vi "test2-TestFilterJKISMStringQueueVI.vi"(8 "error in (no error)":errorcluster, 11 "TestCase in":refnum<class "testcase-CSMManagementAPI.lvclass">) -> (0 "error out":errorcluster, 3 "TestCase out":refnum<class "testcase-CSMManagementAPI.lvclass">)   [LabVIEW 2017, in "testcase-CSMManagementAPI.lvclass"]
uses:
  testcase-CSMManagementAPI.lvclass
  src/user.lib/_NEVSTOP/Communicable State Machine(CSM)/AdvanceAPI/CSM - Revert Arguments-Safe String.vi
  src/user.lib/_NEVSTOP/Communicable State Machine(CSM)/_Shared/Trim Single-line Text.vi
  src/user.lib/_NEVSTOP/Communicable State Machine(CSM)/AdvanceAPI/CSM - Make String Arguments Safe.vi
  src/user.lib/_NEVSTOP/Communicable State Machine(CSM)/AdvanceAPI/CSM - Break Down Multiple States String.vi
  src/user.lib/_NEVSTOP/Communicable State Machine(CSM)/AdvanceAPI/CSM - Compact Multiple States.vi
  src/user.lib/_NEVSTOP/Communicable State Machine(CSM)/AdvanceAPI/CSM - Keywords.vi
  src/user.lib/_NEVSTOP/Communicable State Machine(CSM)/_Polymophic/CSM - Filter Interrupt Broadcasts.vi
  src/user.lib/_NEVSTOP/Communicable State Machine(CSM)/_Polymophic/CSM - Filter Status Broadcasts.vi
  src/user.lib/_NEVSTOP/Communicable State Machine(CSM)/_Polymophic/CSM - Filter Broadcasts.vi
  src/user.lib/_NEVSTOP/Communicable State Machine(CSM)/_Polymophic/CSM - Filter Sync Messages.vi
  src/user.lib/_NEVSTOP/Communicable State Machine(CSM)/_Polymophic/CSM - Filter Async without Reply Messages.vi
  src/user.lib/_NEVSTOP/Communicable State Machine(CSM)/_Polymophic/CSM - Filter Async Messages.vi
  src/user.lib/_NEVSTOP/Communicable State Machine(CSM)/_Polymophic/CSM - Filter Messges.vi
  src/user.lib/_NEVSTOP/Communicable State Machine(CSM)/_Polymophic/CSM - Filter Local States.vi
  src/user.lib/_NEVSTOP/Communicable State Machine(CSM)/_Polymophic/CSM - Filter Duplicated Lines.vi
  src/user.lib/_NEVSTOP/Communicable State Machine(CSM)/AdvanceAPI/CSM - Filter Messages to Non-Existing Modules.vi
  <vilib>/addons/_JKI Toolkits/VI Tester/TestCase.llb/TestCase.lvclass
  src/user.lib/_NEVSTOP/Communicable State Machine(CSM)/Communicable State Machine.lvlib
  C:/Program Files (x86)/National Instruments/LabVIEW 2017/vi.lib/addons/_JKI Toolkits/VI Tester/TestCase.llb/TestCase.lvclass
panel:
  out "Filter Duplicate Lines No Comments":bool
  out "Filter Duplicate Lines":bool
  out "Filter Duplicate States(Regardless of async/sync/status/interrupt)":bool
  out "Fiter Interrupt Broadcast":bool
  out "Fiter Status Broadcast":bool
  out "Fiter Broadcasts":bool
  out "Filter Messages To Non Existing CSMs":bool
  out "Filter Sync Messages":bool
  out "Filter Async Messages Without Reply":bool
  out "Filter Async Messages":bool
  out "Filter All Messages":bool
  out "Fiter Local States":bool
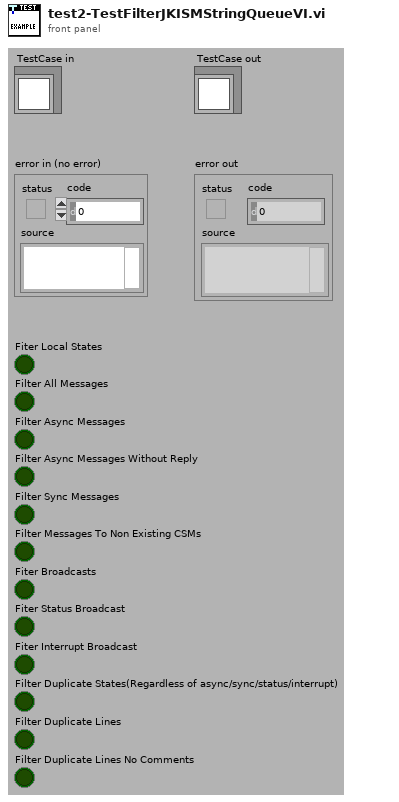
[diagram p1: front panel]
types:
  T1 = enum32{"Invalid", "Standard", "Closed", "Hidden", "Minimized", "Maximized"}
  T2 = enum32{"invalid app kind", "Development System", "Run Time System", "Student Edition", "Embedded LabVIEW", "Evaluation", "Custom"}
  T3 = typedef "Communicable State Machine.lvlib/_CSM_Response Source Message.ctl" = cluster{"‘State":string, "’Arguments":string, "’Error":errorcluster}
  T4 = cluster{"Current VI Reference":refnum<vi>, "Close Panel on Exit?":bool}
  T5 = cluster{"Core":cluster{"Current VI Reference":refnum<vi>, "Close Panel on Exit?":bool}, "Your Boolean data":bool, "Your string data":string}
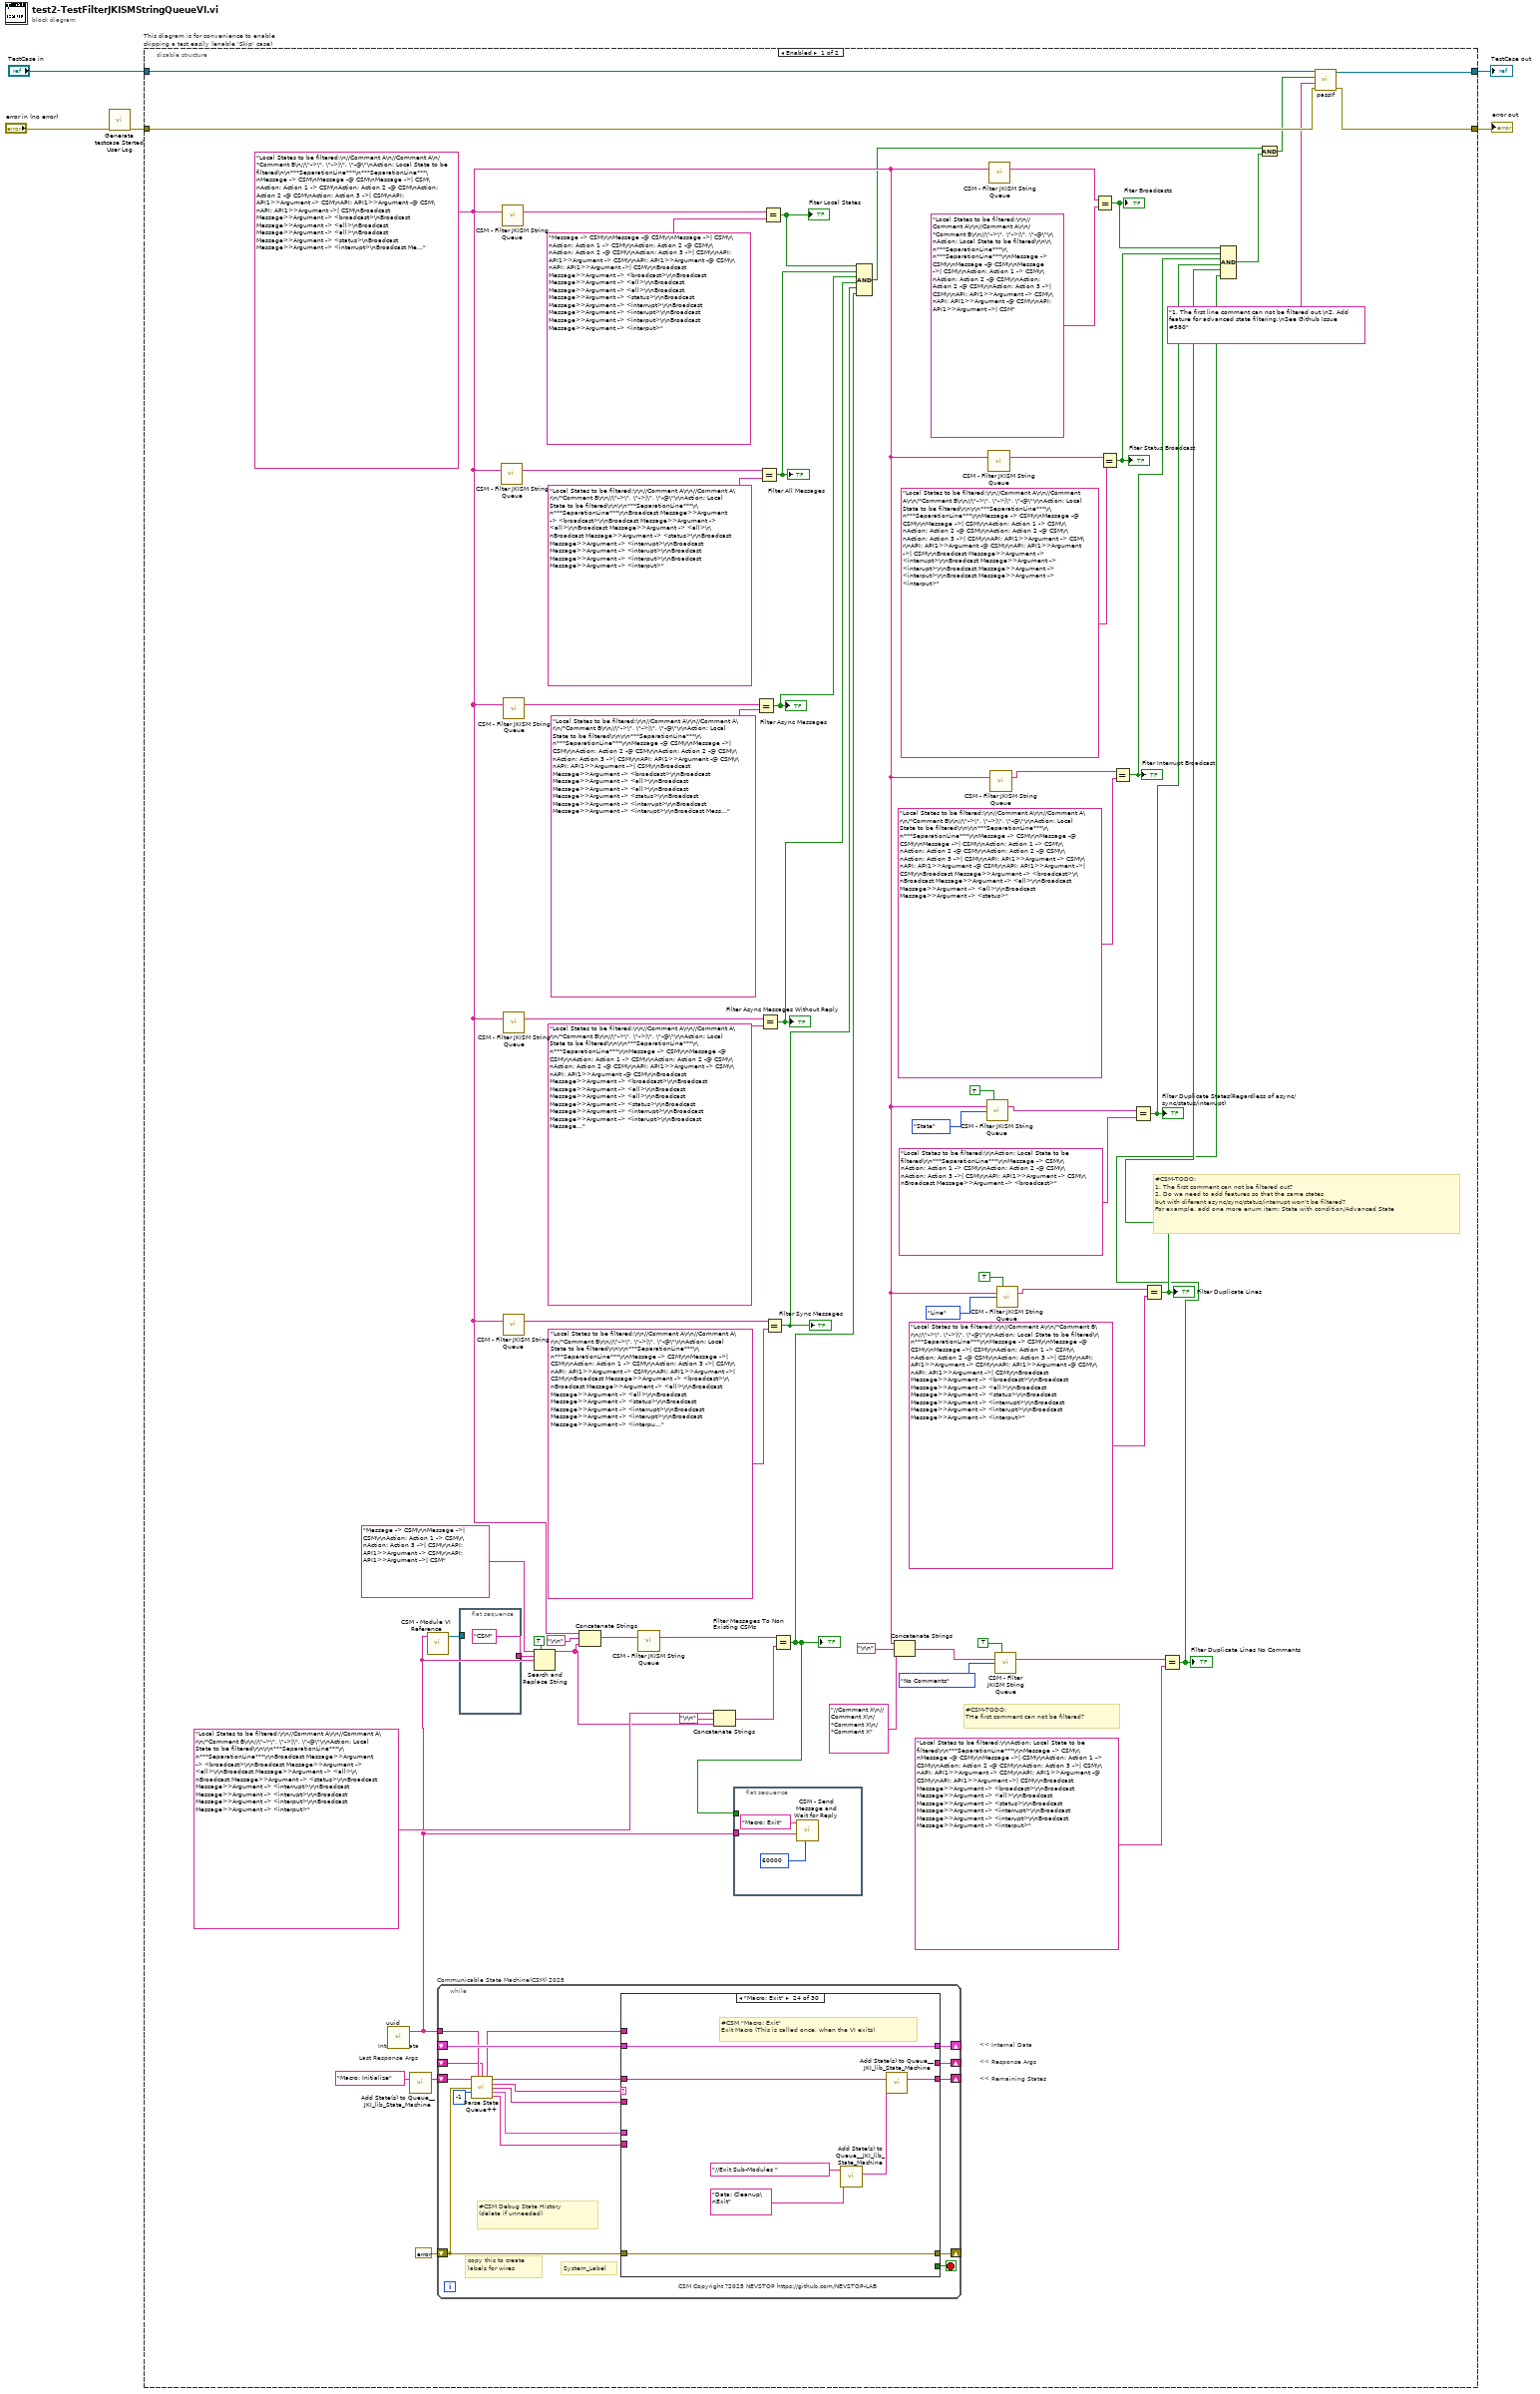
[diagram p0: block diagram]
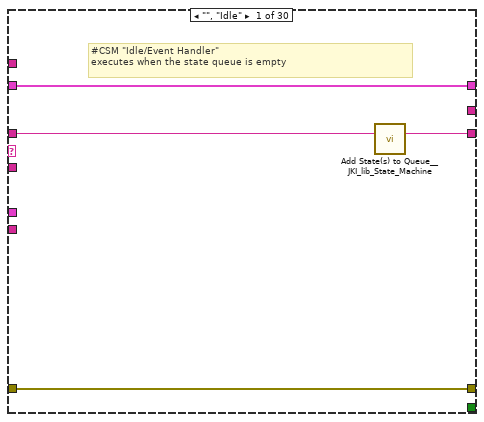
[diagram p2: hidden frame]
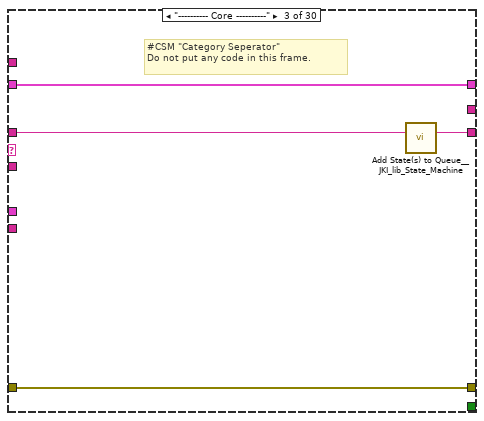
[diagram p4: hidden frame]
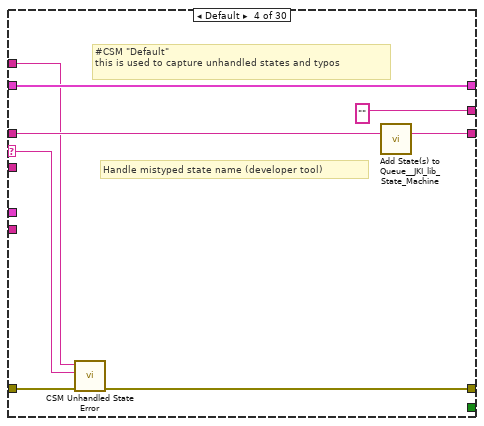
[diagram p5: hidden frame]
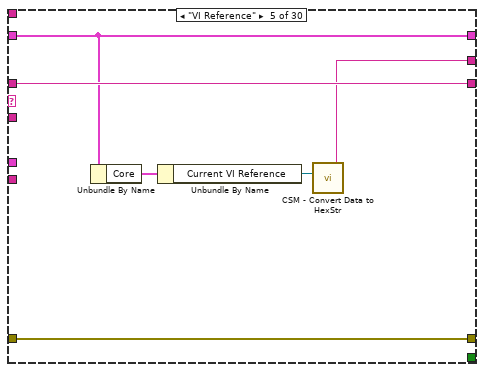
[diagram p6: hidden frame]
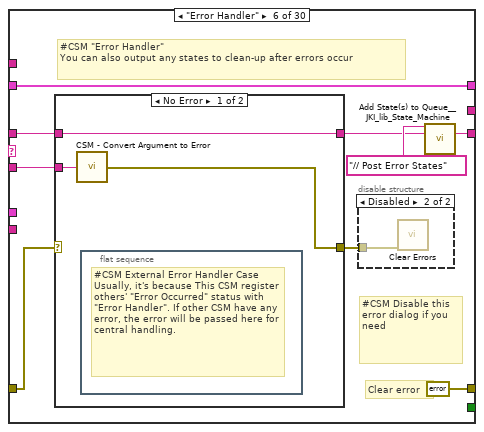
[diagram p7: hidden frame]
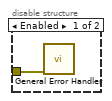
[diagram p8: hidden frame]
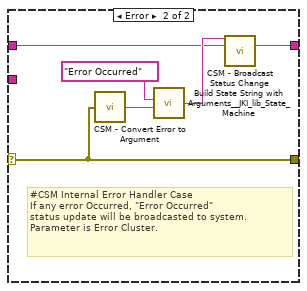
[diagram p9: hidden frame]
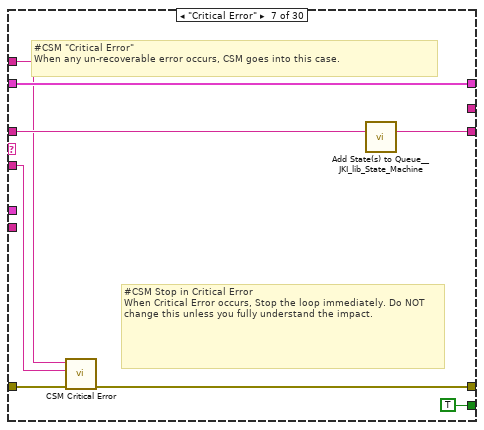
[diagram p10: hidden frame]
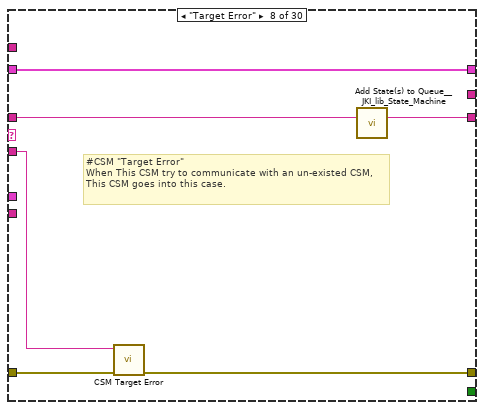
[diagram p11: hidden frame]
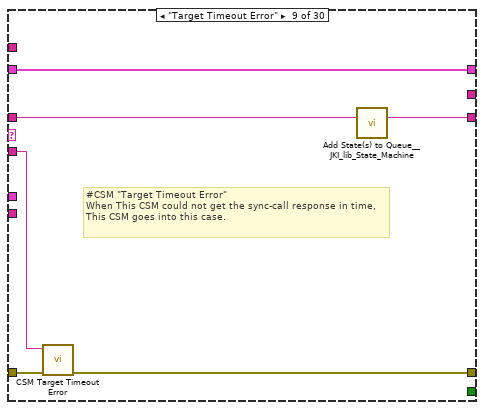
[diagram p12: hidden frame]
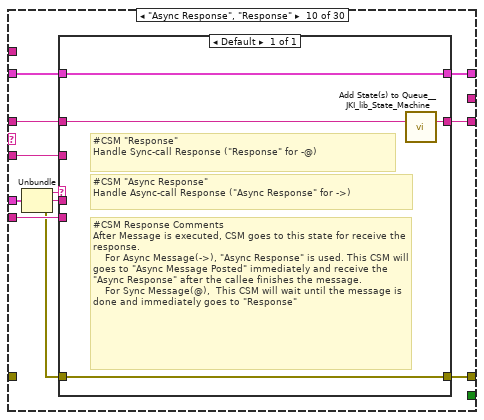
[diagram p13: hidden frame]
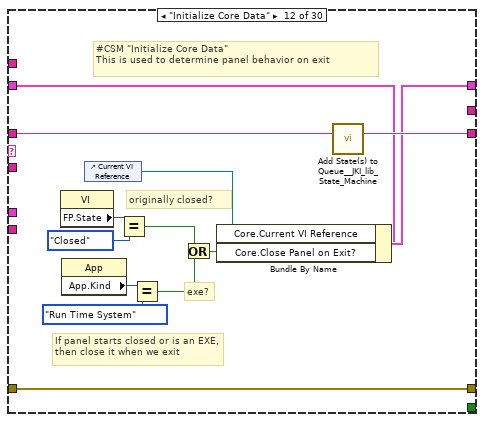
[diagram p15: hidden frame]
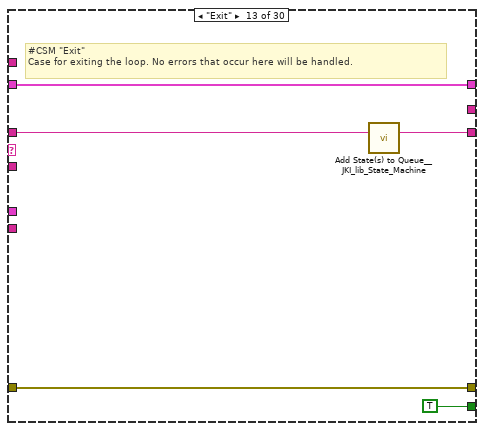
[diagram p16: hidden frame]
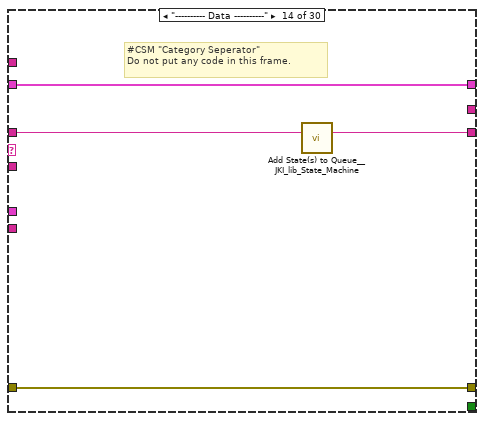
[diagram p17: hidden frame]
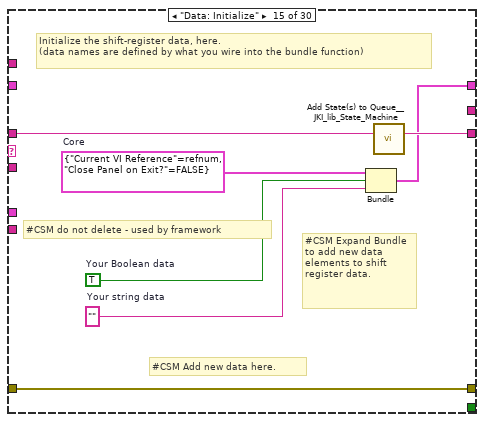
[diagram p18: hidden frame]
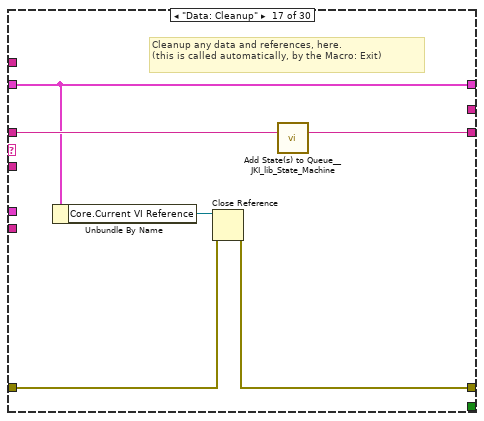
[diagram p20: hidden frame]
diagram:
  n1 = call "Generate testcase Started User Log.vi"("Error In"="error in (no error)") -> ("error out"=w1:errorcluster)  [unwired: 10 in]
  n2 = disable-structure "This diagram is for convenience to enable skipping a test easily (enable 'Skip' case)" shown="Enabled" {
    disable-tunnel: "TestCase in" -> [w32 w354]
    disable-tunnel: [w33 w352] -> w2
    disable-tunnel: [w30 w353] -> w4
    disable-tunnel: w1 -> [w31 w351]
    frame Enabled {
      w38 = "Local States to be filtered:\n//Comment A\n//Comment A\n/*Comment B\n//\"->\", \"->|\", \"-@\"\nAction: Local State to be filtered\n\n***SeparationLine***\n***SeparationLine***\nMessage -> CSM\nMessage -@ CSM\nMessage ->| CSM\nAction: Action 1 -> CSM\nAction: Action 2 -@ CSM\nAction: Action 2 -@ CSM\nAction: Action 3 ->| CSM\nAPI: API1>>Argument -> CSM\nAPI: API1>>Argument -@ CSM\nAPI: API1>>Argument ->| CSM\nBroadcast Message>>Argument -> <broadcast>\nBroadcast Message>>Argument -> <all>\nBroadcast Message>>Argument -> <all>\nBroadcast Message>>Argument -> <status>\nBroadcast Message>>Argument -> <interrupt>\nBroadcast Message>>Argument -> <interupt>\nBroadcast Message>>Argument -> <interput>\nBroadcast Message>>Argument -> <interput>" ("States In")
      # "Last Response Args"
      # "Internal Data"
      # "<< Internal Data"
      # "<< Response Args"
      # "<< Remaining States"
      # "#CSM-TODO:\nTHe first comment can not be filtered?"
      # "#CSM-TODO:\n1. The first comment can not be filtered out?\n2. Do we need to add features so that the same states \nbut with diferent async/sync/status/interrupt won't be filtered?\nFor example, add one more enum item: State with condition/Advanced State"
      n3 = call "uuid.vi"() -> ("UUID"=w7:string)  [unwired: 11 in]
      n4 = call <vilib>:"Add State(s) to Queue__JKI_lib_State_Machine.vi"("State(s) in (\"\")"="Macro: Initialize" ("Init State(\"Macro: Initialize\")")) -> ("States Out"=w11:string)  [unwired: 14 in]
      n5 = call "CSM - Module VI Reference.vi"("CSM Name"=w7) -> ("CSM Module VIRef"=w8:refnum<vi>)  [unwired: 9 in, 1 out]
      n6 = while "Communicable State Machine(CSM) 2025" {
        shift-right: [w88] -> _
        shift-left: _ -> [w87]
        shift-right: [w91] -> _
        shift-left: errorcluster {"status"=FALSE, "code"=0, "source"=""} ("error out") -> [w86]
        shift-right: [w90] -> _
        shift-left: w11 -> [w92]
        tunnel: w7 -> [w84]
        shift-right: [w85] -> _
        shift-left: _ -> [w78]
        stop <- w89 stop-if-true
        # "#CSM Debug State History\n(delete if unneeded)"
        # "copy this to create labels for wires"
        # "System_Label"
        # "CSM Copyright ?2025 NEVSTOP https://github.com/NEVSTOP-LAB"
        n7 = call "Parse State Queue++.vi"("State Queue"=w92, "Name (\"\" to Use UUID)"=w84, "Response Arguments"=w78, "Previous Error"=w86, "Dequeue (1 ms)"=-1 ("Timeout")) -> ("Name Used"=w79:string, "Remaining States"=w93:string, "Current State"=w83:string, "Arguments"=w82:string, "Additional Information"=w81:T3, "Source CSM"=w80:string)  [unwired: 5 in]
        n8 = case shown="\"Macro: Exit\"" w83 {
          selector: w83 -> [_ _ _ w107 _ _ _ _ _ _ _ _ _ _ _ _ _ _ _ _ _ _ _ _ _ _ _ _ _ _]
          tunnel: w93 -> [w94 w99 w104 w111 w117 w123 w144 w150 w156 w164 w175 w189 w194 w198 w205 w207 w214 w218 w222 w228 w243 w312 w317 w324 w326 w330 w335 w342 w346 w350]
          tunnel: w82 -> [_ _ _ _ _ w122 w140 w149 w154 w163 _ _ _ _ _ _ _ _ _ w223 w237 _ _ _ _ _ w333 _ _ _]
          tunnel: w87 -> [w95 w98 w101 w109 w116 w126 w145 w151 w157 w166 w174 w182 w192 w195 _ w206 w209 w215 w220 w226 w239 w309 w314 w321 w325 w329 w334 w339 w343 w347]
          tunnel: [w96 w100 w102 w105 w118 errorcluster {"status"=FALSE, "code"=0, "source"=""} ("error out") w141 w147 w153 w169 w176 w186 w191 w196 w202 w208 w210 w216 w219 w224 w240 w310 w315 w322 w327 w331 w336 w340 w344 w348] -> w91
          tunnel: w86 -> [w96 w100 w102 w112 w118 w124 w146 w148 w155 _ w176 w186 w191 w196 w202 w208 w211 w216 w219 w225 w241 w310 w315 w322 w327 w331 w336 w340 w344 w348]
          tunnel: [w97 w99 w103 w110 w117 w119 w143 w152 w158 w165 w175 w188 w193 w197 w204 w207 w213 w217 w221 w227 w242 w311 w316 w323 w326 w330 w335 w341 w345 w349] -> w90
          tunnel: [_ _ _ _ _ _ TRUE _ _ _ _ _ TRUE _ _ _ _ _ _ _ _ _ _ _ _ _ _ _ _ _] -> w89
          tunnel: [w95 w98 w101 w109 w116 w126 w145 w151 w157 w167 w174 w187 w192 w195 w203 w206 w209 w215 w220 w226 w239 w309 w314 w321 w325 w329 w334 w339 w343 w347] -> w88
          tunnel: w80 -> [_ _ _ _ _ _ _ _ _ w161 _ _ _ _ _ _ _ _ _ _ _ _ _ _ _ _ _ _ _ _]
          tunnel: w81 -> [_ _ _ _ _ _ _ _ _ w168 _ _ _ _ _ _ _ _ _ _ _ _ _ _ _ _ _ _ _ _]
          tunnel: [_ _ _ "" w113 _ _ _ _ _ _ _ _ _ _ _ _ _ _ _ _ _ _ _ _ "API1 Response" w332 _ _ _] -> w85
          tunnel: w79 -> [_ _ _ w106 _ _ w139 _ _ _ _ _ _ _ _ _ _ _ _ _ _ _ _ _ _ _ _ _ _ _]
          frame "", "Idle" {
            # "#CSM \"Idle/Event Handler\"\nexecutes when the state queue is empty"
            n9 = call <vilib>:"Add State(s) to Queue__JKI_lib_State_Machine.vi"("State(s) in (\"\")"=w94) -> ("States Out"=w97:string)  [unwired: 14 in]
          }
          frame "CSM Documentation" {
            # "#CSM README FIRST\n\nCommunicable State Machine(CSM) is a LabVIEW application framework that builds upon JKI State Machine(JKISM). It follows the pattern of JKISM and extends the keywords to describe message communication between modules, including concepts such as Sync-Message, Async-Message, Subscription/Unsubscription of status - essential elements for creating reusable code modules. For more information, please visit the CSM wiki: https://nevstop-lab.github.io/CSM-Wiki/\n\nFor instructions on JKI State Machine, visit: http://jki.net/state-machine/\nFor information about CSM, visit: https://github.com/NEVSTOP-LAB"
            # "#CSM \"Documentation\"\nCase for holding CSM Documenation"
          }
          frame "---------- Core ----------" {
            # "#CSM \"Category Seperator\"\nDo not put any code in this frame."
            n10 = call <vilib>:"Add State(s) to Queue__JKI_lib_State_Machine.vi"("State(s) in (\"\")"=w104) -> ("States Out"=w103:string)  [unwired: 14 in]
          }
          frame Default {
            # "#CSM \"Default\"\nthis is used to capture unhandled states and typos"
            # "Handle mistyped state name (developer tool)"
            n11 = call "CSM Unhandled State Error.vi"("error in (no error)"=w112, "Undefined State"=w107, "CSM Name"=w106) -> ("error out"=w105:errorcluster)  [unwired: 8 in]
            n12 = call <vilib>:"Add State(s) to Queue__JKI_lib_State_Machine.vi"("State(s) in (\"\")"=w111) -> ("States Out"=w110:string)  [unwired: 14 in]
          }
          frame "VI Reference" {
            n13 = Unbundle By Name(w116) -> ("Core"=w115:T4)
            n14 = Unbundle By Name(w115) -> ("Current VI Reference"=w114:refnum<vi>)
            n15 = call "CSM - Convert Data to HexStr.vi"("Variant"=w114) -> ("HEX String (0-9,A-F)"=w113:string)  [unwired: 8 in]
          }
          frame "Error Handler" {
            # "#CSM Disable this error dialog if you need"
            # "#CSM \"Error Handler\"\nYou can also output any states to clean-up after errors occur"
            # "Clear error"
            n16 = case shown="No Error" w124 {
              selector: w124 -> [_ w133]
              tunnel: [w132 w135] -> w120
              tunnel: w123 -> [w132 w134]
              tunnel: w122 -> [w131 _]
              tunnel: [w130 w133] -> w125
              frame No Error {
                n17 = call "CSM - Convert Argument to Error.vi"("Argument"=w131) -> ("Error"=w130:errorcluster)  [unwired: 4 in]
                n18 = flat-sequence {
                  frame #0 {
                    # "#CSM External Error Handler Case\nUsually, it's because This CSM register others' \"Error Occurred\" status with \"Error Handler\". If other CSM have any error, the error will be passed here for central handling."
                  }
                }
              }
              frame Error {
                # "#CSM Internal Error Handler Case \nIf any error Occurred, \"Error Occurred\" \nstatus update will be broadcasted to system.\nParameter is Error Cluster."
                n19 = call "CSM - Convert Error to Argument.vi"("Error"=w133) -> ("Argument"=w137:string)  [unwired: 4 in]
                n20 = call <vilib>:"Build State String with Arguments__JKI_lib_State_Machine.vi"("Arguments (\"\")"=w137, "State"="Error Occurred" ("Status with Arguments")) -> ("State with Arguments"=w136:string)  [unwired: 4 in]
                n21 = call "CSM - Broadcast Status Change.vi"("Status With Arguments"=w136, "State Queue"=w134) -> ("Remaining States"=w135:string)  [unwired: 13 in]
              }
            }
            n22 = disable-structure shown="Disabled" {
              disable-tunnel: w125 -> [w128 w129]
              frame Enabled {
                n23 = call <vilib>:"General Error Handler.vi"("error in (no error)"=w128) -> ()  [unwired: 10 in, 5 out]
              }
              frame Disabled {
                n24 = call <vilib>:"Clear Errors.vi"("error in (no error)"=w129) -> ()  [unwired: 5 in, 2 out]
              }
            }
            n25 = call <vilib>:"Add State(s) to Queue__JKI_lib_State_Machine.vi"("State(s) in Front (\"\")"="// Post Error States", "State(s) in (\"\")"=w120) -> ("States Out"=w119:string)  [unwired: 13 in]
          }
          frame "Critical Error" {
            # "#CSM Stop in Critical Error\nWhen Critical Error occurs, Stop the loop immediately. Do NOT change this unless you fully understand the impact."
            # "#CSM \"Critical Error\"\nWhen any un-recoverable error occurs, CSM goes into this case."
            n26 = call "CSM Critical Error.vi"("error in (no error)"=w146, "Arugments (As Reason)"=w140, "CSM Name"=w139) -> ("error out"=w141:errorcluster)  [unwired: 8 in]
            n27 = call <vilib>:"Add State(s) to Queue__JKI_lib_State_Machine.vi"("State(s) in (\"\")"=w144) -> ("States Out"=w143:string)  [unwired: 14 in]
          }
          frame "Target Error" {
            # "#CSM \"Target Error\"\nWhen This CSM try to communicate with an un-existed CSM, This CSM goes into this case."
            n28 = call "CSM Target Error.vi"("error in (no error)"=w148, "Arguments (As CSM Name)"=w149) -> ("error out"=w147:errorcluster)  [unwired: 9 in]
            n29 = call <vilib>:"Add State(s) to Queue__JKI_lib_State_Machine.vi"("State(s) in (\"\")"=w150) -> ("States Out"=w152:string)  [unwired: 14 in]
          }
          frame "Target Timeout Error" {
            # "#CSM \"Target Timeout Error\"\nWhen This CSM could not get the sync-call response in time, This CSM goes into this case."
            n30 = call "CSM Target Timeout Error.vi"("error in (no error)"=w155, "Arguments (As CSM Name)"=w154) -> ("error out"=w153:errorcluster)  [unwired: 9 in]
            n31 = call <vilib>:"Add State(s) to Queue__JKI_lib_State_Machine.vi"("State(s) in (\"\")"=w156) -> ("States Out"=w158:string)  [unwired: 14 in]
          }
          frame "Async Response", "Response" {
            n32 = Unbundle(w168) -> ("‘State"=w162:string, "’Arguments"=w160:string, "’Error"=w159:errorcluster)
            n33 = case shown="Default" w162 {
              tunnel: [w173] -> w169
              tunnel: w159 -> [w173]
              tunnel: [w172] -> w167
              tunnel: w166 -> [w172]
              tunnel: [w170] -> w165
              tunnel: w164 -> [w171]
              tunnel: w163 -> [_]
              tunnel: w161 -> [_]
              tunnel: w160 -> [_]
              frame Default {
                # "#CSM Response Comments\nAfter Message is executed, CSM goes to this state for receive the response.\n    For Async Message(->), \"Async Response\" is used. This CSM will goes to \"Async Message Posted\" immediately and receive the \"Async Response\" after the callee finishes the message.\n    For Sync Message(@),  This CSM will wait until the message is done and immediately goes to \"Response\""
                # "#CSM \"Async Response\"\nHandle Async-call Response (\"Async Response\" for ->)"
                # "#CSM \"Response\"\nHandle Sync-call Response (\"Response\" for -@)"
                n34 = call <vilib>:"Add State(s) to Queue__JKI_lib_State_Machine.vi"("State(s) in (\"\")"=w171) -> ("States Out"=w170:string)  [unwired: 14 in]
              }
            }
          }
          frame "Async Message Posted" {
            # "#CSM \"Async Message Posted\"\nAfter Async Message is posted (-> or ->| ), CSM goes to this state for post-action.\nYou can use Argument - State to tell which Async Message is called."
          }
          frame "Initialize Core Data" {
            # "#CSM \"Initialize Core Data\"\nThis is used to determine panel behavior on exit"
            # "originally closed?"
            # "exe?"
            # "If panel starts closed or is an EXE, then close it when we exit"
            n35 = property class="VI"() -> ("FP.State"=w179:T1)  [unwired: 2 in, 2 out]
            n36 = property class="App"() -> ("App.Kind"=w185:T2)  [unwired: 2 in, 2 out]
            n37 = control-ref of="Current VI Reference"() -> (w180:refnum<vi>)
            n38 = Equal?(x=w179, y=T1."Closed" ("Front Panel Window:State")) -> (x = y?=w177:bool)
            n39 = Equal?(x=w185, y=T2."Run Time System" ("Application:Kind")) -> (x = y?=w183:bool)
            n40 = Or(x=w177, y=w183) -> (x .or. y?=w181:bool)
            n41 = Bundle By Name(cluster=w182, "Core.Current VI Reference"=w180, "Core.Close Panel on Exit?"=w181) -> (w187:T5)
            n42 = call <vilib>:"Add State(s) to Queue__JKI_lib_State_Machine.vi"("State(s) in (\"\")"=w189) -> ("States Out"=w188:string)  [unwired: 14 in]
          }
          frame "Exit" {
            # "#CSM \"Exit\"\nCase for exiting the loop. No errors that occur here will be handled."
            n43 = call <vilib>:"Add State(s) to Queue__JKI_lib_State_Machine.vi"("State(s) in (\"\")"=w194) -> ("States Out"=w193:string)  [unwired: 14 in]
          }
          frame "---------- Data ----------" {
            # "#CSM \"Category Seperator\"\nDo not put any code in this frame."
            n44 = call <vilib>:"Add State(s) to Queue__JKI_lib_State_Machine.vi"("State(s) in (\"\")"=w198) -> ("States Out"=w197:string)  [unwired: 14 in]
          }
          frame "Data: Initialize" {
            w199 = T4 {"Current VI Reference"=refnum, "Close Panel on Exit?"=FALSE}  # Core
            w201 = TRUE  # Your Boolean data
            w200 = ""  # Your string data
            # "#CSM do not delete - used by framework"
            # "#CSM Expand Bundle to add new data elements to shift register data."
            # "#CSM Add new data here."
            # "Initialize the shift-register data, here.\n(data names are defined by what you wire into the bundle function)"
            n45 = Bundle("Core"=w199, "Your Boolean data"=w201, "Your string data"=w200) -> (w203:T5)  [unwired: 1 in]
            n46 = call <vilib>:"Add State(s) to Queue__JKI_lib_State_Machine.vi"("State(s) in (\"\")"=w205) -> ("States Out"=w204:string)  [unwired: 14 in]
          }
          frame "Data: Update Indicators" {
          }
          frame "Data: Cleanup" {
            # "Cleanup any data and references, here.\n(this is called automatically, by the Macro: Exit)"
            n47 = Unbundle By Name(w209) -> ("Core.Current VI Reference"=w212:refnum<vi>)
            n48 = Close Reference(reference=w212, error in (no error)=w211) -> (error out=w210:errorcluster)
            n49 = call <vilib>:"Add State(s) to Queue__JKI_lib_State_Machine.vi"("State(s) in (\"\")"=w214) -> ("States Out"=w213:string)  [unwired: 14 in]
          }
          frame "---------- UI ----------" {
            # "#CSM \"Category Seperator\"\nDo not put any code in this frame."
            n50 = call <vilib>:"Add State(s) to Queue__JKI_lib_State_Machine.vi"("State(s) in (\"\")"=w218) -> ("States Out"=w217:string)  [unwired: 14 in]
          }
          frame "UI: Initialize" {
            # "#CSM \"UI: Initialize\"\nInitialize the User Interface, here.\n(this is called automatically, by the Macro: Init)"
            n51 = call <vilib>:"Add State(s) to Queue__JKI_lib_State_Machine.vi"("State(s) in (\"\")"=w222) -> ("States Out"=w221:string)  [unwired: 14 in]
          }
          frame "UI: Cursor Set" {
            # "#CSM \"UI: Cursor Set\"\nSet and Unset Cursor Busy.\n(Usage: \"UI: Cursor Set >> Busy|Idle\")"
            # "Argument"
            n52 = disable-structure shown="TARGET_TYPE!=Windows" {
              disable-tunnel: w225 -> [w231 w236]
              disable-tunnel: [w230 w236] -> w224
              disable-tunnel: w223 -> [w229 _]
              frame condition #0 (active) {
                n53 = case shown="\"Idle\", Default" w229 {
                  tunnel: w231 -> [w233 w235]
                  tunnel: [w232 w234] -> w230
                  frame "Idle", Default {
                    n54 = call <vilib>:"Unset Busy.vi"("error in (no error)"=w233) -> ("error out"=w232:errorcluster)  [unwired: 10 in]
                  }
                  frame "Busy" {
                    n55 = call <vilib>:"Set Busy.vi"("error in (no error)"=w235) -> ("error out"=w234:errorcluster)  [unwired: 9 in, 1 out]
                  }
                }
              }
              frame condition #1 {
              }
            }
            n56 = call <vilib>:"Add State(s) to Queue__JKI_lib_State_Machine.vi"("State(s) in (\"\")"=w228) -> ("States Out"=w227:string)  [unwired: 14 in]
          }
          frame "UI: Front Panel State" {
            # "#CSM \"UI: Front Panel State\"\nSet Front Panel Open or Closed\n(Usage: \"UI: Front Panel State >> Open|Close\")"
            # "Argument"
            n57 = Unbundle By Name(w239) -> ("Core.Current VI Reference"=w238:refnum<vi>)
            n58 = call <vilib>:"Add State(s) to Queue__JKI_lib_State_Machine.vi"("State(s) in (\"\")"=w243) -> ("States Out"=w242:string)  [unwired: 14 in]
            n59 = case shown="\"Close\", \"Closed\"" w237 {
              tunnel: w241 -> [w249 w264 w275 w288 w301]
              tunnel: [w251 w265 w277 w290 w303] -> w240
              tunnel: w238 -> [w250 w262 w276 w289 w302]
              frame "Open", "Standard", Default {
                w244 = T1."Standard" ("State")
                n60 = property class="VI"(reference=w250, error in=w249) -> (reference out=w247:refnum<vi>, error out=w248:errorcluster, "FP.State"=w246:T1)
                n61 = Not Equal?(x=w246, y=w244) -> (x != y?=w245:bool)
                n62 = case shown="True" w245 {
                  tunnel: [w255 w257] -> w251
                  tunnel: w248 -> [w254 w257]
                  tunnel: w247 -> [w253 _]
                  tunnel: w244 -> [w252 _]
                  frame True {
                    n63 = invoke class="VI" method="FP.Open"(reference=w253, error in=w254, "Activate"=TRUE, "State"=w252) -> (error out=w255:errorcluster)  [unwired: 1 in, 4 out]
                  }
                  frame False {
                  }
                }
              }
              frame "Close", "Closed" {
                n64 = property class="VI"(reference=w262, error in=w264) -> (reference out=w261:refnum<vi>, error out=w263:errorcluster, "FP.State"=w259:T1)
                n65 = Not Equal?(x=w259, y=T1."Closed" ("Front Panel Window:State")) -> (x != y?=w258:bool)
                n66 = case shown="False" w258 {
                  tunnel: [w266 w269] -> w265
                  tunnel: w263 -> [w266 w268]
                  tunnel: w261 -> [_ w267]
                  frame False {
                  }
                  frame True {
                    n67 = invoke class="VI" method="FP.Close"(reference=w267, error in=w268) -> (error out=w269:errorcluster)  [unwired: 1 in, 2 out]
                  }
                }
              }
              frame "Hidden", "Hide" {
                w270 = T1."Hidden" ("State")
                n68 = property class="VI"(reference=w276, error in=w275) -> (reference out=w273:refnum<vi>, error out=w274:errorcluster, "FP.State"=w272:T1)
                n69 = Not Equal?(x=w272, y=w270) -> (x != y?=w271:bool)
                n70 = case shown="True" w271 {
                  tunnel: [w281 w282] -> w277
                  tunnel: w274 -> [w280 w282]
                  tunnel: w273 -> [w279 _]
                  tunnel: w270 -> [w278 _]
                  frame True {
                    n71 = invoke class="VI" method="FP.Open"(reference=w279, error in=w280, "State"=w278) -> (error out=w281:errorcluster)  [unwired: 2 in, 4 out]
                  }
                  frame False {
                  }
                }
              }
              frame "Minimize", "Minimized" {
                w283 = T1."Minimized" ("State")
                n72 = property class="VI"(reference=w289, error in=w288) -> (reference out=w286:refnum<vi>, error out=w287:errorcluster, "FP.State"=w285:T1)
                n73 = Not Equal?(x=w285, y=w283) -> (x != y?=w284:bool)
                n74 = case shown="True" w284 {
                  tunnel: [w294 w295] -> w290
                  tunnel: w287 -> [w293 w295]
                  tunnel: w286 -> [w292 _]
                  tunnel: w283 -> [w291 _]
                  frame True {
                    n75 = invoke class="VI" method="FP.Open"(reference=w292, error in=w293, "State"=w291) -> (error out=w294:errorcluster)  [unwired: 2 in, 4 out]
                  }
                  frame False {
                  }
                }
              }
              frame "Maximize", "Maximized" {
                w296 = T1."Maximized" ("State")
                n76 = property class="VI"(reference=w302, error in=w301) -> (reference out=w299:refnum<vi>, error out=w300:errorcluster, "FP.State"=w298:T1)
                n77 = Not Equal?(x=w298, y=w296) -> (x != y?=w297:bool)
                n78 = case shown="True" w297 {
                  tunnel: [w307 w308] -> w303
                  tunnel: w300 -> [w306 w308]
                  tunnel: w299 -> [w305 _]
                  tunnel: w296 -> [w304 _]
                  frame True {
                    n79 = invoke class="VI" method="FP.Open"(reference=w305, error in=w306, "State"=w304) -> (error out=w307:errorcluster)  [unwired: 2 in, 4 out]
                  }
                  frame False {
                  }
                }
              }
            }
          }
          frame "---------- Macro ----------" {
            # "#CSM \"Category Seperator\"\nDo not put any code in this frame."
            n80 = call <vilib>:"Add State(s) to Queue__JKI_lib_State_Machine.vi"("State(s) in (\"\")"=w312) -> ("States Out"=w311:string)  [unwired: 14 in]
          }
          frame "Macro: Initialize" {
            # "#CSM \"Macro: Initialize\"\nInitialization Macro (This is called once, when the VI starts)"
            n81 = call <vilib>:"Add State(s) to Queue__JKI_lib_State_Machine.vi"("State(s) in Front (\"\")"="Data: Initialize\nInitialize Core Data\nData: Update Indicators", "State(s) in (\"\")"=w317) -> ("States Out"=w316:string)  [unwired: 13 in]
          }
          frame "Macro: Exit" {
            # "#CSM \"Macro: Exit\"\nExit Macro (This is called once, when the VI exits)"
            n82 = call <vilib>:"Add State(s) to Queue__JKI_lib_State_Machine.vi"("State(s) in Front (\"\")"="//Exit Sub-Modules ", "State(s) at Back (\"\")"="Data: Cleanup\nExit") -> ("States Out"=w319:string)  [unwired: 13 in]
            n83 = call <vilib>:"Add State(s) to Queue__JKI_lib_State_Machine.vi"("State(s) in Front (\"\")"=w319, "State(s) in (\"\")"=w324) -> ("States Out"=w323:string)  [unwired: 13 in]
          }
          frame "---------- API ----------" {
            # "#CSM \"Category Seperator\"\nDo not put any code in this frame."
          }
          frame "API: API1" {
            # "#CSM API Example\nCopy/Rename this case for your own API"
            # "#CSM Response\nConnect this to return the response of your API"
            # "#CSM >> Msg/Rep's CSM >>\nIf you need to tell who triggered this state , use this string. If it's this case itself, this string is \"\"."
            # "#CSM >> Arguments >>\nDeal with the parameter if any"
          }
          frame "API: API2" {
            # "#CSM API Example\nCopy/Rename this case for your own API"
            # "unpack Hex String  to Variant\nif complex parameter is needed."
            n84 = call "CSM - Convert HexStr to Data.vi"("HEX String"=w333) -> ()  [unwired: 7 in, 2 out]
            n85 = disable-structure shown="Disabled" {
              disable-tunnel: [w337 "API2 Response"] -> w332
              frame Disabled {
                # "pack variant to hexstr \nif complex response is needed."
                # "complex Response"
                n86 = call "CSM - Convert Data to HexStr.vi"() -> ("HEX String (0-9,A-F)"=w337:string)  [unwired: 9 in]
              }
              frame Enabled {
              }
            }
          }
          frame "---------- Action ----------" {
            # "#CSM \"Category Seperator\"\nDo not put any code in this frame."
            n87 = call <vilib>:"Add State(s) to Queue__JKI_lib_State_Machine.vi"("State(s) in (\"\")"=w342) -> ("States Out"=w341:string)  [unwired: 14 in]
          }
          frame "Action: action1" {
            # "#CSM \"Internal State\"\nThis category is used for holding internal states"
            n88 = call <vilib>:"Add State(s) to Queue__JKI_lib_State_Machine.vi"("State(s) in (\"\")"=w346) -> ("States Out"=w345:string)  [unwired: 14 in]
          }
          frame "Action: action2" {
            # "#CSM \"Internal State\"\nThis category is used for holding internal states"
            n89 = call <vilib>:"Add State(s) to Queue__JKI_lib_State_Machine.vi"("State(s) in (\"\")"=w350) -> ("States Out"=w349:string)  [unwired: 14 in]
          }
        }
      }
      n90 = flat-sequence {
        tunnel: ["CSM" ("search string")] -> w61
        tunnel: w8 -> [_]
        frame #0 {
        }
      }
      n91 = call-poly "CSM - Filter JKISM String Queue.vi"("States In"=w38) -> ("States Out"=w70:string)  [unwired: 14 in]
      n92 = call-poly "CSM - Filter JKISM String Queue.vi"("States In"=w38) -> ("States Out"=w72:string)  [unwired: 14 in]
      n93 = call-poly "CSM - Filter JKISM String Queue.vi"("States In"=w38) -> ("States Out"=w64:string)  [unwired: 14 in]
      n94 = call-poly "CSM - Filter JKISM String Queue.vi"("States In"=w38) -> ("States Out"=w68:string)  [unwired: 14 in]
      n95 = call-poly "CSM - Filter JKISM String Queue.vi"("States In"=w38) -> ("States Out"=w66:string)  [unwired: 14 in]
      n96 = Search and Replace String(replace all?=TRUE ("replace all? (F)"), input string="Message -> CSM\r\nMessage ->| CSM\r\nAction: Action 1 -> CSM\r\nAction: Action 3 ->| CSM\r\nAPI: API1>>Argument -> CSM\r\nAPI: API1>>Argument ->| CSM", search string=w61, replace string=w7) -> (result string=w57:string)  [unwired: 4 in, 3 out]
      n97 = Concatenate Strings(w38, "\r\n", w57) -> (w59:string)
      n98 = call-poly "CSM - Filter JKISM String Queue.vi"("States In"=w59) -> ("States Out"=w56:string)  [unwired: 14 in]
      n99 = Concatenate Strings("Local States to be filtered:\r\n//Comment A\r\n//Comment A\r\n/*Comment B\r\n//\"->\", \"->|\", \"-@\"\r\nAction: Local State to be filtered\r\n\r\n***SeparationLine***\r\n***SeparationLine***\r\nBroadcast Message>>Argument -> <broadcast>\r\nBroadcast Message>>Argument -> <all>\r\nBroadcast Message>>Argument -> <all>\r\nBroadcast Message>>Argument -> <status>\r\nBroadcast Message>>Argument -> <interrupt>\r\nBroadcast Message>>Argument -> <interupt>\r\nBroadcast Message>>Argument -> <interput>\r\nBroadcast Message>>Argument -> <interput>" ("States Out"), "\r\n", w57) -> (w55:string)
      n100 = flat-sequence {
        tunnel: w7 -> [w75]
        tunnel: w6 -> [_]
        frame #0 {
          n101 = call "CSM - Send Message and Wait for Reply.vi"("Response Timeout (-2 Using Global Settings)"=60000, "Target Module"=w75, "State"="Macro: Exit") -> ()  [unwired: 6 in, 3 out]
        }
      }
      n102 = Equal?(x=w68, y="Local States to be filtered:\r\n//Comment A\r\n//Comment A\r\n/*Comment B\r\n//\"->\", \"->|\", \"-@\"\r\nAction: Local State to be filtered\r\n\r\n***SeparationLine***\r\n***SeparationLine***\r\nMessage -@ CSM\r\nMessage ->| CSM\r\nAction: Action 2 -@ CSM\r\nAction: Action 2 -@ CSM\r\nAction: Action 3 ->| CSM\r\nAPI: API1>>Argument -@ CSM\r\nAPI: API1>>Argument ->| CSM\r\nBroadcast Message>>Argument -> <broadcast>\r\nBroadcast Message>>Argument -> <all>\r\nBroadcast Message>>Argument -> <all>\r\nBroadcast Message>>Argument -> <status>\r\nBroadcast Message>>Argument -> <interrupt>\r\nBroadcast Message>>Argument -> <interupt>\r\nBroadcast Message>>Argument -> <interput>\r\nBroadcast Message>>Argument -> <interput>" ("States In")) -> (x = y?=w27:bool)
      "Filter Async Messages" <- w27
      n103 = Equal?(x=w70, y="Local States to be filtered:\r\n//Comment A\r\n//Comment A\r\n/*Comment B\r\n//\"->\", \"->|\", \"-@\"\r\nAction: Local State to be filtered\r\n\r\n***SeparationLine***\r\n***SeparationLine***\r\nBroadcast Message>>Argument -> <broadcast>\r\nBroadcast Message>>Argument -> <all>\r\nBroadcast Message>>Argument -> <all>\r\nBroadcast Message>>Argument -> <status>\r\nBroadcast Message>>Argument -> <interrupt>\r\nBroadcast Message>>Argument -> <interupt>\r\nBroadcast Message>>Argument -> <interput>\r\nBroadcast Message>>Argument -> <interput>" ("States In")) -> (x = y?=w28:bool)
      "Filter All Messages" <- w28
      n104 = Equal?(x=w66, y="Local States to be filtered:\r\n//Comment A\r\n//Comment A\r\n/*Comment B\r\n//\"->\", \"->|\", \"-@\"\r\nAction: Local State to be filtered\r\n\r\n***SeparationLine***\r\n***SeparationLine***\r\nMessage -> CSM\r\nMessage -@ CSM\r\nAction: Action 1 -> CSM\r\nAction: Action 2 -@ CSM\r\nAction: Action 2 -@ CSM\r\nAPI: API1>>Argument -> CSM\r\nAPI: API1>>Argument -@ CSM\r\nBroadcast Message>>Argument -> <broadcast>\r\nBroadcast Message>>Argument -> <all>\r\nBroadcast Message>>Argument -> <all>\r\nBroadcast Message>>Argument -> <status>\r\nBroadcast Message>>Argument -> <interrupt>\r\nBroadcast Message>>Argument -> <interupt>\r\nBroadcast Message>>Argument -> <interput>\r\nBroadcast Message>>Argument -> <interput>" ("States Out")) -> (x = y?=w26:bool)
      "Filter Async Messages Without Reply" <- w26
      n105 = Equal?(x=w72, y="Message -> CSM\r\nMessage -@ CSM\r\nMessage ->| CSM\r\nAction: Action 1 -> CSM\r\nAction: Action 2 -@ CSM\r\nAction: Action 2 -@ CSM\r\nAction: Action 3 ->| CSM\r\nAPI: API1>>Argument -> CSM\r\nAPI: API1>>Argument -@ CSM\r\nAPI: API1>>Argument ->| CSM\r\nBroadcast Message>>Argument -> <broadcast>\r\nBroadcast Message>>Argument -> <all>\r\nBroadcast Message>>Argument -> <all>\r\nBroadcast Message>>Argument -> <status>\r\nBroadcast Message>>Argument -> <interrupt>\r\nBroadcast Message>>Argument -> <interupt>\r\nBroadcast Message>>Argument -> <interput>\r\nBroadcast Message>>Argument -> <interput>" ("States Out")) -> (x = y?=w29:bool)
      "Fiter Local States" <- w29
      n106 = Equal?(x=w64, y="Local States to be filtered:\r\n//Comment A\r\n//Comment A\r\n/*Comment B\r\n//\"->\", \"->|\", \"-@\"\r\nAction: Local State to be filtered\r\n\r\n***SeparationLine***\r\n***SeparationLine***\r\nMessage -> CSM\r\nMessage ->| CSM\r\nAction: Action 1 -> CSM\r\nAction: Action 3 ->| CSM\r\nAPI: API1>>Argument -> CSM\r\nAPI: API1>>Argument ->| CSM\r\nBroadcast Message>>Argument -> <broadcast>\r\nBroadcast Message>>Argument -> <all>\r\nBroadcast Message>>Argument -> <all>\r\nBroadcast Message>>Argument -> <status>\r\nBroadcast Message>>Argument -> <interrupt>\r\nBroadcast Message>>Argument -> <interupt>\r\nBroadcast Message>>Argument -> <interput>\r\nBroadcast Message>>Argument -> <interput>" ("States Out")) -> (x = y?=w25:bool)
      "Filter Sync Messages" <- w25
      n107 = Equal?(x=w56, y=w55) -> (x = y?=w6:bool)
      "Filter Messages To Non Existing CSMs" <- w6
      n108 = Compound Arithmetic op=AND(w29, w28, w27, w26, w25, w6) -> (w18:bool)
      n109 = Concatenate Strings(w38, "\r\n", "//Comment X\n//Comment X\n/*Comment X\n/*Comment X" ("States Out")) -> (w35:string)
      n110 = call-poly "CSM - Filter JKISM String Queue.vi"("Keep First Matched? (T)"=TRUE, "States In"=w38, "Option"=enum16{"State", "No Comments", "Line"}."State") -> ("States Out"=w46:string)  [unwired: 12 in]
      n111 = call-poly "CSM - Filter JKISM String Queue.vi"("States In"=w38) -> ("States Out"=w52:string)  [unwired: 14 in]
      n112 = call-poly "CSM - Filter JKISM String Queue.vi"("States In"=w38) -> ("States Out"=w54:string)  [unwired: 14 in]
      n113 = call-poly "CSM - Filter JKISM String Queue.vi"("States In"=w38) -> ("States Out"=w50:string)  [unwired: 14 in]
      n114 = call-poly "CSM - Filter JKISM String Queue.vi"("Keep First Matched? (T)"=TRUE, "States In"=w35, "Option"=enum16{"State", "No Comments", "Line"}."No Comments") -> ("States Out"=w37:string)  [unwired: 12 in]
      n115 = call-poly "CSM - Filter JKISM String Queue.vi"("Keep First Matched? (T)"=TRUE, "States In"=w38, "Option"=enum16{"State", "No Comments", "Line"}."Line") -> ("States Out"=w42:string)  [unwired: 12 in]
      n116 = Equal?(x=w54, y="Local States to be filtered:\r\n//Comment A\r\n//Comment A\r\n/*Comment B\r\n//\"->\", \"->|\", \"-@\"\r\nAction: Local State to be filtered\r\n\r\n***SeparationLine***\r\n***SeparationLine***\r\nMessage -> CSM\r\nMessage -@ CSM\r\nMessage ->| CSM\r\nAction: Action 1 -> CSM\r\nAction: Action 2 -@ CSM\r\nAction: Action 2 -@ CSM\r\nAction: Action 3 ->| CSM\r\nAPI: API1>>Argument -> CSM\r\nAPI: API1>>Argument -@ CSM\r\nAPI: API1>>Argument ->| CSM" ("States Out")) -> (x = y?=w24:bool)
      "Fiter Broadcasts" <- w24
      n117 = Equal?(x=w52, y="Local States to be filtered:\r\n//Comment A\r\n//Comment A\r\n/*Comment B\r\n//\"->\", \"->|\", \"-@\"\r\nAction: Local State to be filtered\r\n\r\n***SeparationLine***\r\n***SeparationLine***\r\nMessage -> CSM\r\nMessage -@ CSM\r\nMessage ->| CSM\r\nAction: Action 1 -> CSM\r\nAction: Action 2 -@ CSM\r\nAction: Action 2 -@ CSM\r\nAction: Action 3 ->| CSM\r\nAPI: API1>>Argument -> CSM\r\nAPI: API1>>Argument -@ CSM\r\nAPI: API1>>Argument ->| CSM\r\nBroadcast Message>>Argument -> <interrupt>\r\nBroadcast Message>>Argument -> <interupt>\r\nBroadcast Message>>Argument -> <interput>\r\nBroadcast Message>>Argument -> <interput>" ("States Out")) -> (x = y?=w23:bool)
      "Fiter Status Broadcast" <- w23
      n118 = Equal?(x=w50, y="Local States to be filtered:\r\n//Comment A\r\n//Comment A\r\n/*Comment B\r\n//\"->\", \"->|\", \"-@\"\r\nAction: Local State to be filtered\r\n\r\n***SeparationLine***\r\n***SeparationLine***\r\nMessage -> CSM\r\nMessage -@ CSM\r\nMessage ->| CSM\r\nAction: Action 1 -> CSM\r\nAction: Action 2 -@ CSM\r\nAction: Action 2 -@ CSM\r\nAction: Action 3 ->| CSM\r\nAPI: API1>>Argument -> CSM\r\nAPI: API1>>Argument -@ CSM\r\nAPI: API1>>Argument ->| CSM\r\nBroadcast Message>>Argument -> <broadcast>\r\nBroadcast Message>>Argument -> <all>\r\nBroadcast Message>>Argument -> <all>\r\nBroadcast Message>>Argument -> <status>" ("States Out")) -> (x = y?=w22:bool)
      "Fiter Interrupt Broadcast" <- w22
      n119 = Equal?(x=w46, y="Local States to be filtered:\r\nAction: Local State to be filtered\r\n***SeparationLine***\r\nMessage -> CSM\r\nAction: Action 1 -> CSM\r\nAction: Action 2 -@ CSM\r\nAction: Action 3 ->| CSM\r\nAPI: API1>>Argument -> CSM\r\nBroadcast Message>>Argument -> <broadcast>" ("States Out")) -> (x = y?=w21:bool)
      "Filter Duplicate States(Regardless of async/sync/status/interrupt)" <- w21
      n120 = Equal?(x=w42, y="Local States to be filtered:\r\n//Comment A\r\n/*Comment B\r\n//\"->\", \"->|\", \"-@\"\r\nAction: Local State to be filtered\r\n***SeparationLine***\r\nMessage -> CSM\r\nMessage -@ CSM\r\nMessage ->| CSM\r\nAction: Action 1 -> CSM\r\nAction: Action 2 -@ CSM\r\nAction: Action 3 ->| CSM\r\nAPI: API1>>Argument -> CSM\r\nAPI: API1>>Argument -@ CSM\r\nAPI: API1>>Argument ->| CSM\r\nBroadcast Message>>Argument -> <broadcast>\r\nBroadcast Message>>Argument -> <all>\r\nBroadcast Message>>Argument -> <status>\r\nBroadcast Message>>Argument -> <interrupt>\r\nBroadcast Message>>Argument -> <interupt>\r\nBroadcast Message>>Argument -> <interput>" ("States Out")) -> (x = y?=w20:bool)
      "Filter Duplicate Lines" <- w20
      n121 = Equal?(x=w37, y="Local States to be filtered:\r\nAction: Local State to be filtered\r\n***SeparationLine***\r\nMessage -> CSM\r\nMessage -@ CSM\r\nMessage ->| CSM\r\nAction: Action 1 -> CSM\r\nAction: Action 2 -@ CSM\r\nAction: Action 3 ->| CSM\r\nAPI: API1>>Argument -> CSM\r\nAPI: API1>>Argument -@ CSM\r\nAPI: API1>>Argument ->| CSM\r\nBroadcast Message>>Argument -> <broadcast>\r\nBroadcast Message>>Argument -> <all>\r\nBroadcast Message>>Argument -> <status>\r\nBroadcast Message>>Argument -> <interrupt>\r\nBroadcast Message>>Argument -> <interupt>\r\nBroadcast Message>>Argument -> <interput>" ("States Out")) -> (x = y?=w19:bool)
      "Filter Duplicate Lines No Comments" <- w19
      n122 = Compound Arithmetic op=AND(w24, w23, w22, w21, w20, w19) -> (w17:bool)
      n123 = And(x=w18, y=w17) -> (x .and. y?=w16:bool)
      n124 = call-dynamic "passIf.vi"("error in (no error)"=w31, "message (\"\")"="1. The first line comment can not be filtered out.\n2. Add feature for advanced state filtering.\nSee Github Issue #580" ("message (\"\")"), "pass"=w16, "TestCase in"=w32) -> ("error out"=w30:errorcluster, "TestCase out"=w33:refnum<class "testcase-CSMManagementAPI.lvclass">)  [unwired: 6 in]
    }
    frame Disabled {
      # "skip test result while test is under development"
      n125 = call <vilib>:"skip.vi"("error in (no error)"=w351, "TestCase in"=w354) -> ("error out"=w353:errorcluster, "TestCase out"=w352:refnum<class "testcase-CSMManagementAPI.lvclass">)  [unwired: 8 in]
    }
  }
  "error out" <- w4
  "TestCase out" <- w2
